vi "STRING_POT_CAL 2016.vi"(6 "Sensor Cluster":T1, 7 "Array in":refnum<k24>[](array[refnum]), 8 "error in (no error)":errorcluster, 9 "Descriptions":string[](array[string]), 11 "string_pot_slope_IN":dbl=51.35 format="%.2f") -> (0 "error out":errorcluster, 3 "string_pot_slope_OUT":dbl=51.35 format="%.2f", 4 "Sensor Cluster 2":T1, 5 "Array out":refnum<k24>[](array[refnum]))   [LabVIEW 2016]
uses:
  C:/Program Files (x86)/National Instruments/LabVIEW 2016/vi.lib/ULx/ULx_LV.dll
  controls/MCC DAQ Readings.ctl
  Global_SIM_switch.vi
  Kpro Globals.vi
panel:
  in  "Calibration \nDistance":dbl=5.0 format="%#_13g"
  out "String Pot \nSlope":dbl=1.7339999675750732 format="%.2f"
  out "delta Distance":dbl
  out "Distance(ft)":dbl format="%.2f"
  in  "stop":bool
  in  "start":bool
  # "STRING POTENTIOMETER CALIBRATION"
  # "Hold string pot wire at 5' above the string pot body.\nPress start."
  # "Slowly lower the string pot wire.\nPress Stop when t he string pot wire is fully retracted."
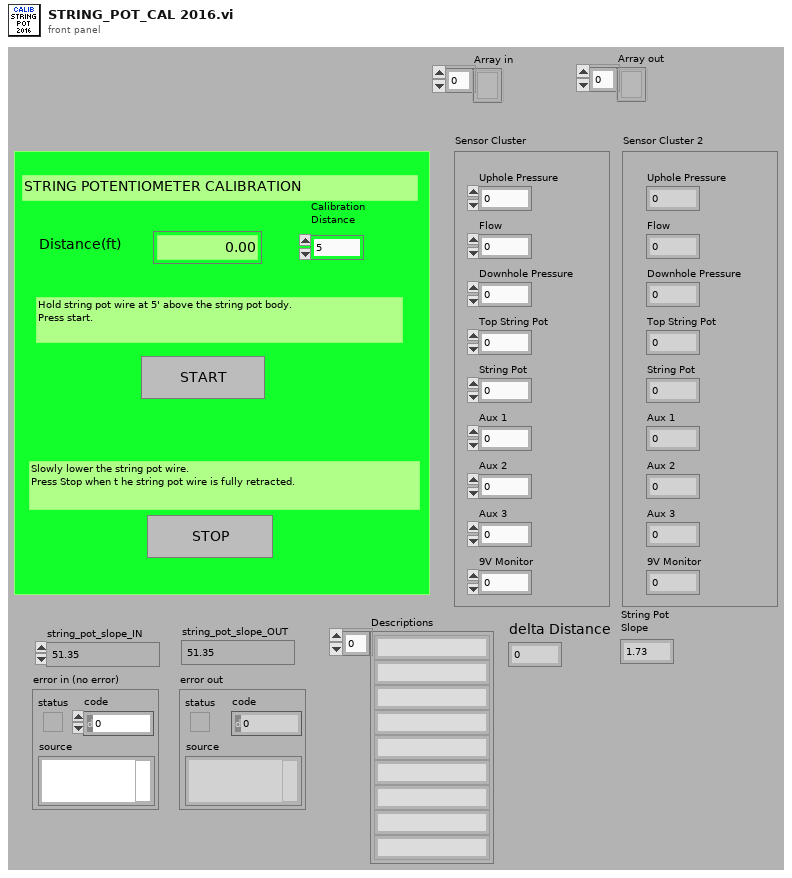
[diagram p1: front panel]
types:
  T1 = typedef "MCC DAQ Readings.ctl" = cluster{"Uphole Pressure":dbl, "Flow":dbl, "Downhole Pressure":dbl, "Top String Pot":dbl, "String Pot":dbl, "Aux 1":dbl, "Aux 2":dbl, "Aux 3":dbl, "9V Monitor":dbl}
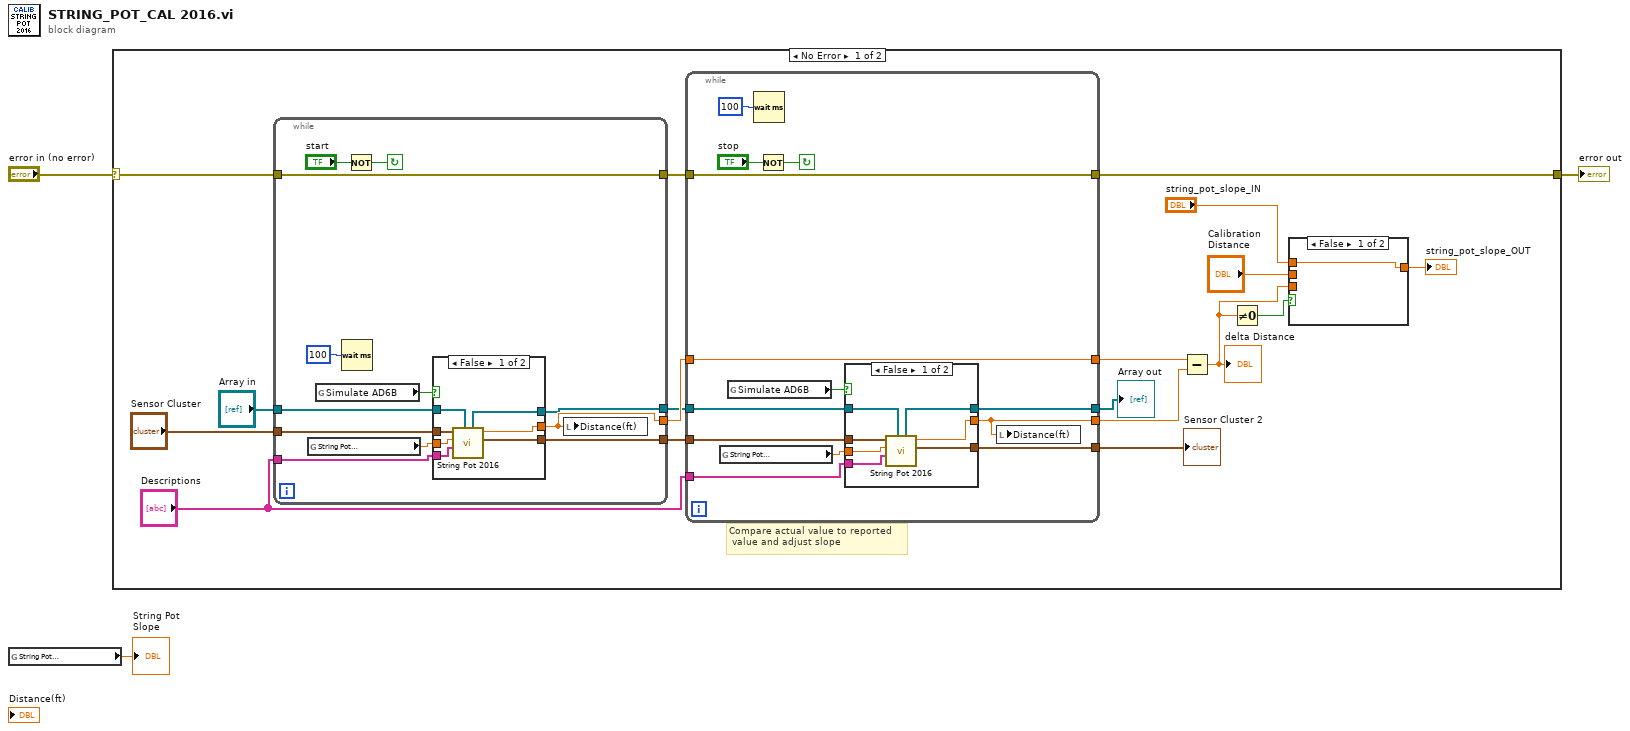
[diagram p0: block diagram]
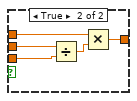
[diagram p2: hidden frame]
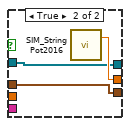
[diagram p3: hidden frame]
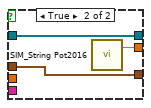
[diagram p4: hidden frame]
diagram:
  n1 = global read "Kpro Globals.vi" "String Pot \nSlope"() -> (→"String Pot \nSlope":dbl)
  n2 = case shown="No Error" "error in (no error)" {
    selector: "error in (no error)" -> [w21 w73]
    tunnel: [w19 w73] -> w3
    frame No Error {
      # "Compare actual value to reported\n value and adjust slope"
      n3 = while {
        tunnel: [w34] -> w16
        tunnel: [w37] -> w20
        tunnel: w21 -> [w37]
        tunnel: "Array in" -> [w33]
        tunnel: "Sensor Cluster" -> [w32]
        tunnel: "Descriptions" -> [w31]
        tunnel: [w30] -> w8
        tunnel: [w29] -> w10
        stop <- w38 continue-if-true
        n4 = global read "Kpro Globals.vi" "String Pot \nSlope"() -> (w28:dbl)
        n5 = global read "Global_SIM_switch.vi" "Simulate AD6B"() -> (w36:bool)
        n6 = Wait (ms)(milliseconds to wait=u32 100) -> ()  [unwired: 1 out]
        n7 = Not(x="start") -> (.not. x?=w38:bool)
        n8 = case shown="False" w36 {
          tunnel: [w46 w49] -> w34
          tunnel: w33 -> [w45 w47]
          tunnel: w32 -> [w44 w48]
          tunnel: w31 -> [w43 _]
          tunnel: [w42 w48] -> w30
          tunnel: [w41 w47] -> w29
          tunnel: w28 -> [w40 _]
          frame False {
            n9 = call "String Pot 2016.vi"("Array in"=w45, "Descriptions"=w43, "String Pot \nSlope"=w40, "Sensor Cluster"=w44) -> ("Sensor Cluster 2"=w42:T1, "Distance (in)"=w46:dbl, "Array out"=w41:refnum<k24>[])  [unwired: 4 in, 1 out]
          }
          frame True {
            n10 = call "SIM_String Pot2016.vi"() -> ("Distance (in)"=w49:dbl)  [unwired: 3 in]
          }
        }
        n11 = local write "Distance(ft)"(w34) -> ()
      }
      n12 = while {
        tunnel: w16 -> [w59]
        tunnel: [w57] -> w15
        tunnel: [w59] -> w14
        tunnel: w20 -> [w60]
        tunnel: [w60] -> w19
        tunnel: "Descriptions" -> [w55]
        tunnel: w10 -> [w54]
        tunnel: [w53] -> w9
        tunnel: w8 -> [w51]
        tunnel: [w50] -> w7
        stop <- w62 continue-if-true
        n13 = global read "Kpro Globals.vi" "String Pot \nSlope"() -> (w52:dbl)
        n14 = global read "Global_SIM_switch.vi" "Simulate AD6B"() -> (w56:bool)
        n15 = Wait (ms)(milliseconds to wait=u32 100) -> ()  [unwired: 1 out]
        n16 = Not(x="stop") -> (.not. x?=w62:bool)
        n17 = case shown="False" w56 {
          tunnel: [w69 w72] -> w57
          tunnel: w54 -> [w68 w70]
          tunnel: w51 -> [w67 w71]
          tunnel: w55 -> [w66 _]
          tunnel: [w65 w71] -> w50
          tunnel: [w64 w70] -> w53
          tunnel: w52 -> [w63 _]
          frame False {
            n18 = call "String Pot 2016.vi"("Array in"=w68, "Descriptions"=w66, "String Pot \nSlope"=w63, "Sensor Cluster"=w67) -> ("Sensor Cluster 2"=w65:T1, "Distance (in)"=w69:dbl, "Array out"=w64:refnum<k24>[])  [unwired: 4 in, 1 out]
          }
          frame True {
            n19 = call "SIM_String Pot2016.vi"() -> ("Distance (in)"=w72:dbl)  [unwired: 3 in]
          }
        }
        n20 = local write "Distance(ft)"(w57) -> ()
      }
      "Sensor Cluster 2" <- w7
      "Array out" <- w9
      n21 = Subtract(x=w14, y=w15) -> (x-y=w5:dbl)
      "delta Distance" <- w5
      n22 = Not Equal To 0?(x=w5) -> (x != 0?=w4:bool)
      n23 = case shown="False" w4 {
        tunnel: "string_pot_slope_IN" -> [w22 w27]
        tunnel: [w22 w26] -> w17
        tunnel: "Calibration \nDistance" -> [_ w24]
        tunnel: w5 -> [_ w23]
        frame False {
        }
        frame True {
          n24 = Divide(x=w24, y=w23) -> (x/y=w25:dbl)
          n25 = Multiply(x=w27, y=w25) -> (x*y=w26:dbl)
        }
      }
      "string_pot_slope_OUT" <- w17
    }
    frame Error {
    }
  }
  "error out" <- w3
